vi "Action.vi"(8 "error in (no error)":errorcluster, 10 "OOQMH in":refnum<class "OOQMH.lvclass">, 11 "PID in":refnum<class "PID.lvclass">) -> (0 "error out":errorcluster, 2 "OOQMH out":refnum<class "OOQMH.lvclass">, 3 "PID out":refnum<class "PID.lvclass">)   [LabVIEW 2024, in "PID Loop.lvlib" / "PID.lvclass"]
uses:
  PID.lvclass
  OOQMH/OOQMH/OOQMH.lvclass
  PID Loop/PID Loop.lvclass
  PID.lvclass/PID.ctl
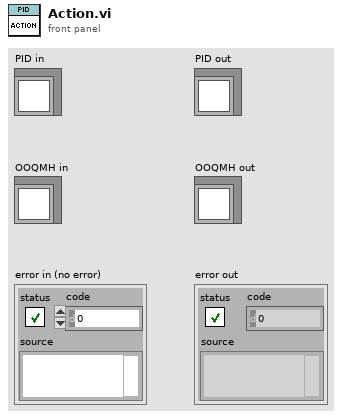
[diagram p1: front panel]
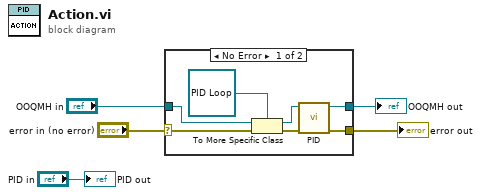
[diagram p0: block diagram]
diagram:
  n1 = case shown="No Error" "error in (no error)" {
    selector: "error in (no error)" -> [w9 w13]
    tunnel: "OOQMH in" -> [w12 w14]
    tunnel: [w10 w14] -> w4
    tunnel: [w7 w13] -> w2
    frame No Error {
      n2 = To More Specific Class(target class=refnum<class "PID Loop.lvclass"> refnum ("PID Loop in"), reference=w12, error in=w9) -> (specific class reference=w11:refnum<class "PID Loop.lvclass">, error out=w8:errorcluster)
      n3 = call-dynamic "PID.vi"("error in (no error)"=w8, "PID Loop in"=w11) -> ("error out"=w7:errorcluster, "PID Loop out"=w10:refnum<class "PID Loop.lvclass">)  [unwired: 8 in]
    }
    frame Error {
    }
  }
  "error out" <- w2
  "OOQMH out" <- w4
  "PID out" <- "PID in"
